vi "Remove_Icon_File.vi"(0 "Files In":path[](array[path])) -> (1 "Files Out":path[](array[path]), 2 "Icon files found?":bool)   [LabVIEW 2012]
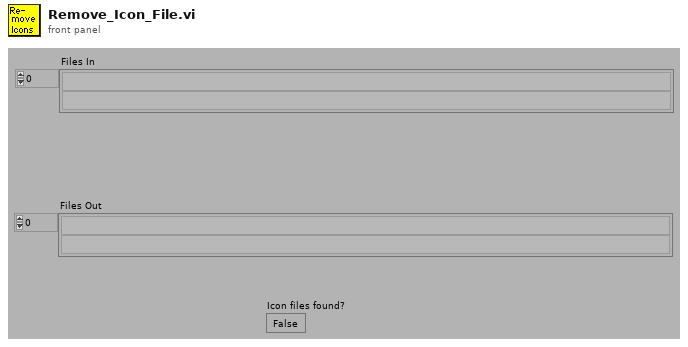
[diagram p1: front panel]
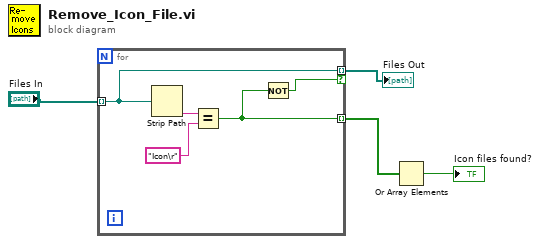
[diagram p0: block diagram]
diagram:
  n1 = for {
    tunnel: "Files In" -> [w7] mode=indexing
    tunnel: [w6] -> w1 mode=indexing
    tunnel: [w7] -> w4 mode=indexing if=w5
    n2 = Strip Path(path=w7) -> (name=w9:string)  [unwired: 1 out]
    n3 = Equal?(x=w9, y="Icon\r") -> (x = y?=w6:bool)
    n4 = Not(x=w6) -> (.not. x?=w5:bool)
  }
  "Files Out" <- w4
  n5 = Or Array Elements(Boolean array=w1) -> (logical OR=→"Icon files found?":bool)
